vi "Create jump table.vi"() -> (3 "Array":dbl[](array[numeric]))   [LabVIEW 2019]
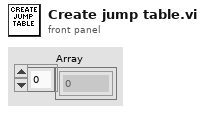
[diagram p1: front panel]
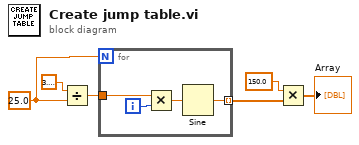
[diagram p0: block diagram]
diagram:
  w1 = 25.0 ("y")
  n1 = Divide(x=3.141592653589793, y=w1) -> (x/y=w3:dbl)
  n2 = for {
    N: w1 -> [_]
    tunnel: w3 -> [w9]
    tunnel: [w7] -> w4 mode=indexing
    i -> [w10]
    n3 = Multiply(x=w9, y=w10) -> (x*y=w8:dbl)
    n4 = Sine(x=w8) -> (sin(x)=w7:dbl)
  }
  n5 = Multiply(x=150.0 ("y"), y=w4) -> (x*y=→"Array":dbl[])
